vi "Execute.vi"(8 "error in (no error)":errorcluster, 9 "System in":refnum<class "System.lvclass">, 10 "Command in":refnum<class "Command.lvclass">, 11 "DM-DFD-StopAtDistance-State in":refnum<class "DM-DFD-StopAtDistance-State.lvclass">) -> (0 "error out":errorcluster, 2 "Next State":refnum<class "State.lvclass">, 3 "DM-DFD-StopAtDistance-State out":refnum<class "DM-DFD-StopAtDistance-State.lvclass">)   [LabVIEW 2013, in "DM-DFD-StopAtDistance-State.lvclass"]
uses:
  DM-DFD-StopAtDistance-State.lvclass
  Commands/Command/Command.lvclass
  Systems/System/System.lvclass
  State/State.lvclass
  Systems/DriveMotors/DriveMotors.lvclass
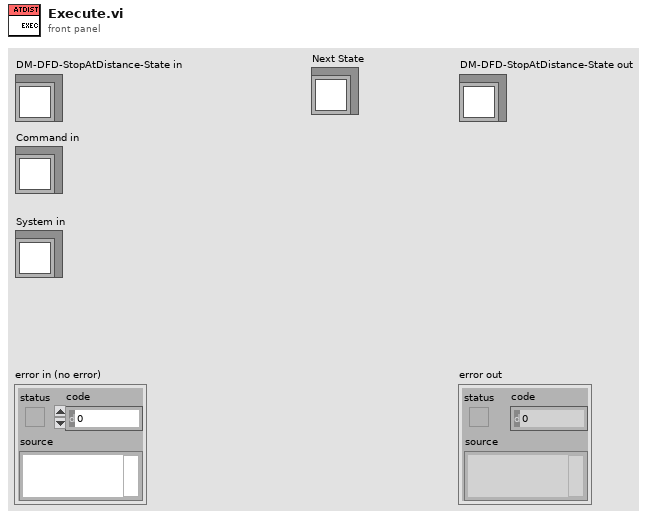
[diagram p1: front panel]
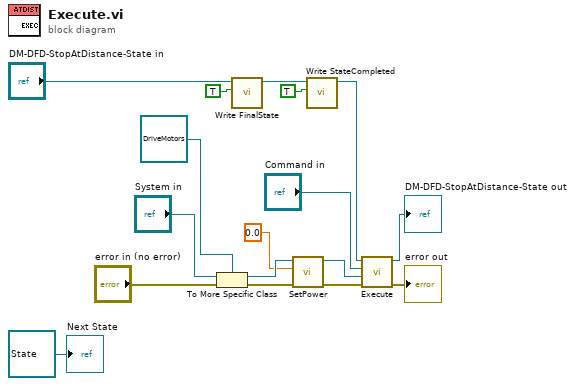
[diagram p0: block diagram]
diagram:
  n1 = To More Specific Class(target class=refnum<class "DriveMotors.lvclass"> refnum ("DriveMotors.lvclass"), reference="System in", error in="error in (no error)") -> (specific class reference=w12:refnum<class "DriveMotors.lvclass">, error out=w9:errorcluster)
  n2 = call-dynamic "Write FinalState.vi"("FinalState"=TRUE, "State in"="DM-DFD-StopAtDistance-State in") -> ("State out"=w6:refnum<class "DM-DFD-StopAtDistance-State.lvclass">)  [unwired: 8 in, 1 out]
  n3 = call-dynamic "SetPower.vi"("error in (no error)"=w9, "MotorPower"=0.0, "DriveMotors in"=w12) -> ("error out"=w8:errorcluster, "DriveMotors out"=w11:refnum<class "DriveMotors.lvclass">)  [unwired: 7 in]
  n4 = call-dynamic "Write StateCompleted.vi"("StateCompleted"=TRUE, "State in"=w6) -> ("State out"=w2:refnum<class "DM-DFD-StopAtDistance-State.lvclass">)  [unwired: 8 in, 1 out]
  n5 = call-parent "Execute.vi"("error in (no error)"=w8, "System in"=w11, "Command in"="Command in", "State in"=w2) -> ("error out"=→"error out":errorcluster, "State out"=→"DM-DFD-StopAtDistance-State out":refnum<class "DM-DFD-StopAtDistance-State.lvclass">)  [unwired: 5 in, 1 out]
  "Next State" <- refnum<class "State.lvclass"> refnum ("State.lvclass")
